vi "Preamble (SubVI).vi"(11 "array in":cdb[](array[numeric])) -> (3 "array out":cdb[](array[numeric]))   [LabVIEW 2015]
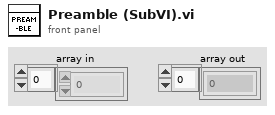
[diagram p1: front panel]
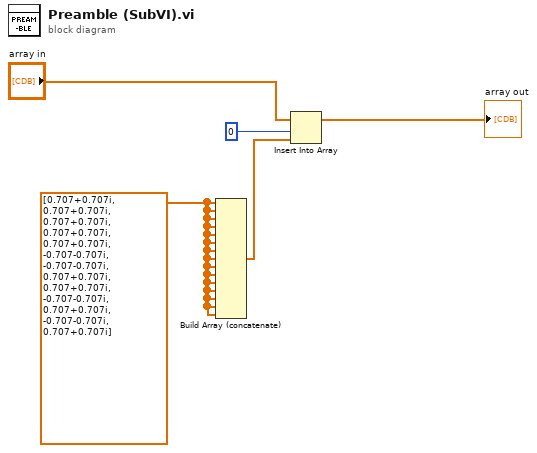
[diagram p0: block diagram]
diagram:
  w1 = cdb[] [0.707+0.707i, 0.707+0.707i, 0.707+0.707i, 0.707+0.707i, 0.707+0.707i, -0.707-0.707i, -0.707-0.707i, 0.707+0.707i, 0.707+0.707i, -0.707-0.707i, 0.707+0.707i, -0.707-0.707i, 0.707+0.707i] ("array 2")
  n1 = Build Array (concatenate)(w1, w1, w1, w1, w1, w1, w1, w1, w1, w1, w1, w1, w1, w1, w1) -> (w5:cdb[])
  n2 = Insert Into Array(array="array in", index=0, new element=w5) -> (→"array out":cdb[])
